vi "Set File Settings.vi"(8 "error in":errorcluster, 9 "Delimiter":enum16{"Tab", "Coma"}(ring), 10 "Save Time Stamp":bool=TRUE) -> (0 "error out":errorcluster)   [LabVIEW 2019, in "ManejoArchivos.lvlib"]
doc: "Set File Settings\n\n_____\nCreated using DQMH Framework: Event Scripter 7.1.0.1490."
uses:
  ManejoArchivos.lvlib
  Set File Settings Argument--cluster.ctl
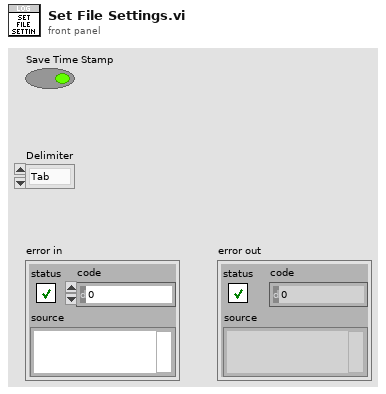
[diagram p1: front panel]
types:
  T1 = typedef "ManejoArchivos.lvlib/Set File Settings Argument--cluster.ctl" = cluster{"Save Time Stamp":bool, "Delimiter":enum16{"Tab", "Coma"}}
  T2 = typedef "ManejoArchivos.lvlib/Request Events--cluster.ctl" = cluster{"Stop Module":refnum<user-event>, "Show Panel":refnum<user-event>, "Hide Panel":refnum<user-event>, "Get Module Execution Status":refnum<user-event>, "Show Diagram":refnum<user-event>, "Set Column Headers":refnum<user-event>, "View File":refnum<user-event>, "Set File Path":refnum<user-event>, "Set File Settings":refnum<user-event>, "Log Data":refnum<user-event>, "Set File Format":refnum<user-event>, "Close File":refnum<user-event>, "Get Number of Columns":refnum<user-event>}
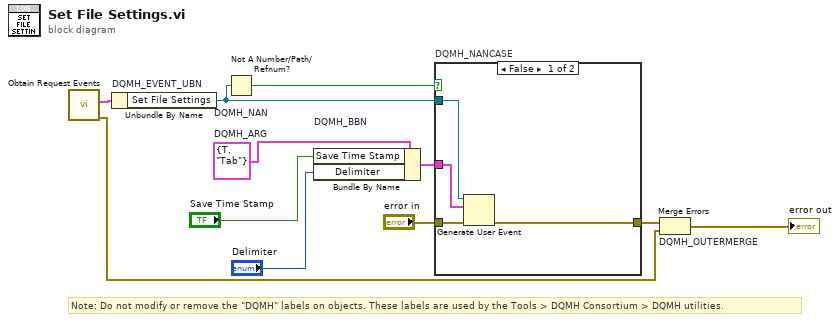
[diagram p0: block diagram]
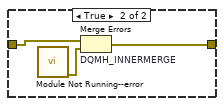
[diagram p2: hidden frame]
diagram:
  w5 = T1 {"Save Time Stamp"=TRUE, "Delimiter"=enum."Tab"}  # DQMH_ARG
  # "Note: Do not modify or remove the \"DQMH\" labels on objects. These labels are used by the Tools > DQMH Consortium > DQMH utilities."
  n1 = call "Obtain Request Events.vi"() -> ("error out"=w2:errorcluster, "ManejoArchivos Request Events"=w1:T2)  [unwired: 10 in]
  n2 = Unbundle By Name "DQMH_EVENT_UBN"(w1) -> ("Set File Settings"=w7:refnum<user-event>)
  n3 = Not A Number/Path/Refnum? "DQMH_NAN"(number/path/refnum=w7) -> (NaN/Path/Refnum?=w8:bool)
  n4 = Bundle By Name "DQMH_BBN"(cluster=w5, "Save Time Stamp"="Save Time Stamp", "Delimiter"="Delimiter") -> (w9:T1)
  n5 = case "DQMH_NANCASE" shown="False" w8 {
    tunnel: "error in" -> [w15 w18]
    tunnel: [w14 w17] -> w6
    tunnel: w7 -> [w13 _]
    tunnel: w9 -> [w12 _]
    frame False {
      n6 = Generate User Event(user event=w13, event data cluster=w12, error in=w15) -> (error out=w14:errorcluster)  [unwired: 1 in, 1 out]
    }
    frame True {
      n7 = call "Module Not Running--error.vi"() -> ("error out"=w16:errorcluster)  [unwired: 11 in]
      n8 = Merge Errors "DQMH_INNERMERGE"(w18, w16) -> (w17:errorcluster)
    }
  }
  n9 = Merge Errors "DQMH_OUTERMERGE"(w6, w2) -> (→"error out":errorcluster)
